vi "_mzData Converter.vi"() -> (0 "Output XML":string)   [LabVIEW 2012]
uses:
  Type/_File Command.ctl
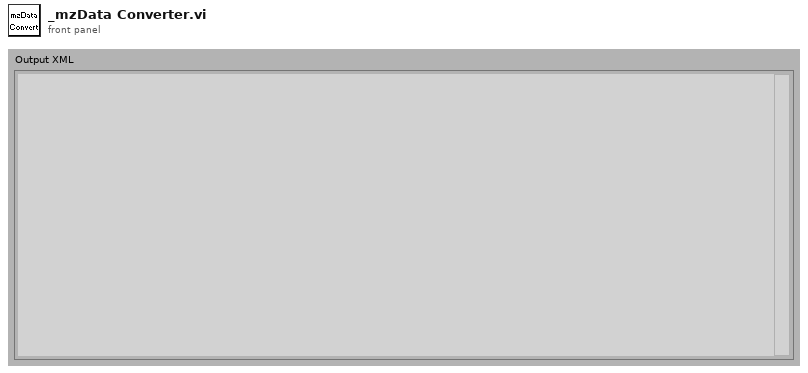
[diagram p1: front panel]
types:
  T1 = enum32{"existing file", "new file", "new or existing file", "existing dir", "new dir", "new or existing dir", "existing file (use LLBs)", "new file (use LLBs)", "new or existing file (use LLBs)", "new or existing file or directory (use LLBs)"}
  T2 = typedef "_File Command.ctl" = enum16{"No Command", "Open", "Open Read", "Write", "Get Spectrum", "Close"}
  T3 = typedef "_XML Expt.ctl" = cluster{"StartT(mS)":i32, "#Cycles":i32, "PauseT(uS)":i32, "ScanType":i32, "Polarity":u8, "FixedMass":dbl, "DelayT(mS)":i32, "Active Ch":T4[], "Mass Range":T5[]}
  T4 = typedef "_XML Lens.ctl" = cluster{"Value":dbl, "ChID":u8}
  T5 = typedef "_Mass Range Property.ctl" = cluster{"Start":dbl, "Stop":dbl, "Step Size":dbl, "Steps":i32, "Dwell":dbl, "Parameters":T6[], "Res":T7}
  T6 = typedef "_Mass Range Parameters.ctl" = cluster{"Name":string, "Ch#":u8, "StartV":dbl, "StopV":dbl, "StepV":dbl, "Index":u8}
  T7 = typedef "_RT Res Type.ctl" = u16
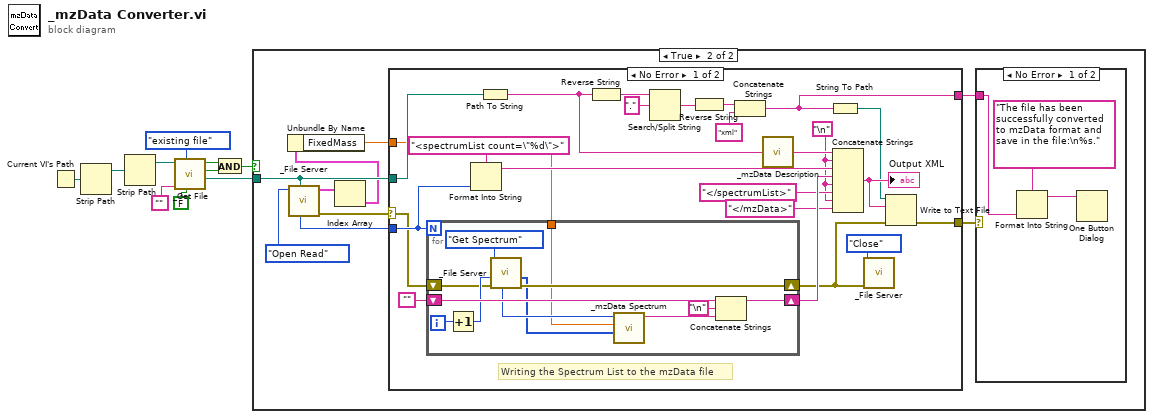
[diagram p0: block diagram]
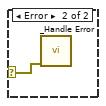
[diagram p3: hidden frame]
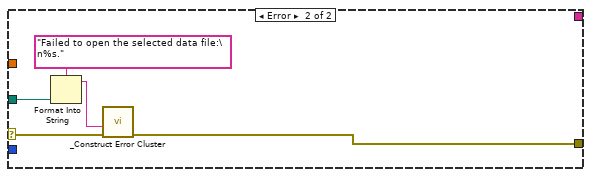
[diagram p4: hidden frame]
diagram:
  n1 = Current VI's Path() -> (path=w7:path)
  n2 = Strip Path(path=w7) -> (stripped path=w8:path)  [unwired: 1 out]
  n3 = Strip Path(path=w8) -> (stripped path=w6:path)  [unwired: 1 out]
  n4 = call "_Get File.vi"("For Write (T)"=FALSE, "select mode (new or existing)"=T1."existing file", "default name"="", "Start Path"=w6) -> ("Seleted File"=w1:path, "Exists"=w3:bool, "Succeeded"=w4:bool)  [unwired: 2 in, 1 out]
  n5 = And(x=w4, y=w3) -> (x .and. y?=w5:bool)
  n6 = case shown="True" w5 {
    tunnel: w1 -> [_ w17]
    frame False {
    }
    frame True {
      n7 = call "_File Server.vi"("file path"=w17, "File Command"=_File_Command."Open Read") -> ("error out"=w18:errorcluster, "AcqMethod 2"=w12:T3[], "Scan# out"=w16:i32)  [unwired: 5 in, 2 out]
      n8 = Index Array(array=w12) -> (element=w11:T3)  [unwired: 1 in]
      n9 = Unbundle By Name(w11) -> ("FixedMass"=w13:dbl)
      n10 = case shown="No Error" w18 {
        selector: w18 -> [w38 w64]
        tunnel: w17 -> [w40 w63]
        tunnel: [w35 w60] -> w15
        tunnel: w16 -> [w39 _]
        tunnel: [w25 _] -> w14
        tunnel: w13 -> [w24 _]
        frame No Error {
          w33 = "\n"
          # "Writing the Spectrum List to the mzData file"
          n11 = for {
            N: w39 -> [_]
            shift-right: [w57] -> w47
            shift-left: "" -> [w59]
            shift-right: [w50] -> w36
            shift-left: w38 -> [w52]
            tunnel: w24 -> [w48]
            i -> [w55]
            n12 = Increment(x=w55) -> (x+1=w53:i32)
            n13 = call "_File Server.vi"("error in (no error)"=w52, "Scan#"=w53, "File Command"=_File_Command."Get Spectrum") -> ("error out"=w50:errorcluster, "Spectrum Out"=w49:u32[], "Scan# out"=w51:i32)  [unwired: 4 in, 2 out]
            n14 = call "_mzData Spectrum.vi"("Spectrum"=w49, "FixedMass (amu)"=w48, "id"=w51) -> ("Output XML"=w56:string)  [unwired: 4 out]
            n15 = Concatenate Strings(w59, "\n", w56) -> (w57:string)
          }
          n16 = Format Into String(format string="<spectrumList count=\"%d\">", w39) -> (resulting string=w42:string)  [unwired: 2 in, 1 out]
          n17 = Path To String(path=w40) -> (string=w32:string)
          n18 = Reverse String(1:w32) -> (0:w31:string)
          n19 = Search/Split String(string=w31, search string/char (-)=".") -> (match + rest of string=w29:string)  [unwired: 3 out]
          n20 = Reverse String(1:w29) -> (0:w28:string)
          n21 = Concatenate Strings(w28, "xml" ("search string/char (-)")) -> (w25:string)
          n22 = call "_mzData Description.vi"("Sample Name"=w32) -> ("Output XML"=w43:string)
          n23 = String To Path(string=w25) -> (path=w26:path)
          n24 = Concatenate Strings(w43, w33, w42, w47, w33, "</spectrumList>", w33, "</mzData>") -> (w34:string)
          "Output XML" <- w34
          n25 = call "_File Server.vi"("error in (no error)"=w36, "File Command"=_File_Command."Close") -> ()  [unwired: 5 in, 5 out]
          n26 = Write to Text File(file (use dialog)=w26, text=w34, error in=w36) -> (error out=w35:errorcluster)  [unwired: 3 out]
        }
        frame Error {
          n27 = Format Into String(format string="Failed to open the selected data file:\n%s.", w63) -> (resulting string=w61:string)  [unwired: 2 in, 1 out]
          n28 = call "_Construct Error Cluster.vi"("error in"=w64, "reason"=w61) -> ("error out"=w60:errorcluster)  [unwired: 2 in, 3 out]
        }
      }
      n29 = case shown="No Error" w15 {
        selector: w15 -> [_ w23]
        tunnel: w14 -> [w22 _]
        frame No Error {
          n30 = Format Into String(format string="The file has been successfully converted to mzData format and save in the file:\n%s.", w22) -> (resulting string=w20:string)  [unwired: 2 in, 1 out]
          n31 = One Button Dialog(message=w20) -> ()  [unwired: 2 out]
        }
        frame Error {
          n32 = call "_Handle Error.vi"("error in (no error)"=w23) -> ()  [unwired: 2 in, 5 out]
        }
      }
    }
  }
